vi "WPI_JoystickMapping.vi"   [LabVIEW 2017]
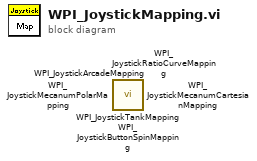
[diagram p0: block diagram]
diagram:
  n1 = call <vilib>:"WPI_JoystickTankMapping.vi"() -> ()  [unwired: 10 in, 2 out]
  n2 = call <vilib>:"WPI_JoystickRatioCurveMapping.vi"() -> ()  [unwired: 10 in, 2 out]
  n3 = call <vilib>:"WPI_JoystickMecanumPolarMapping.vi"() -> ()  [unwired: 8 in, 4 out]
  n4 = call <vilib>:"WPI_JoystickMecanumCartesianMapping.vi"() -> ()  [unwired: 8 in, 4 out]
  n5 = call <vilib>:"WPI_JoystickButtonSpinMapping.vi"() -> ()  [unwired: 10 in, 2 out]
  n6 = call <vilib>:"WPI_JoystickArcadeMapping.vi"() -> ()  [unwired: 10 in, 2 out]
